vi "Load by Identifier.vi"(8 "error in (no error)":errorcluster, 10 "Identifier":string, 11 "InMemoryUserProvider in":refnum<class "InMemoryUserProvider.lvclass">) -> (0 "error out":errorcluster, 2 "User":refnum<class "User.lvclass">, 3 "InMemoryUserProvider out":refnum<class "InMemoryUserProvider.lvclass">)   [LabVIEW 2020, in "HTTP Server.lvlib" / "InMemoryUserProvider.lvclass"]
uses:
  InMemoryUserProvider.lvclass
  InMemoryUserProvider.lvclass/InMemoryUserProvider.ctl
  User/User.lvclass
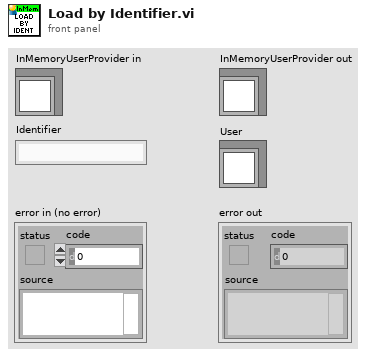
[diagram p1: front panel]
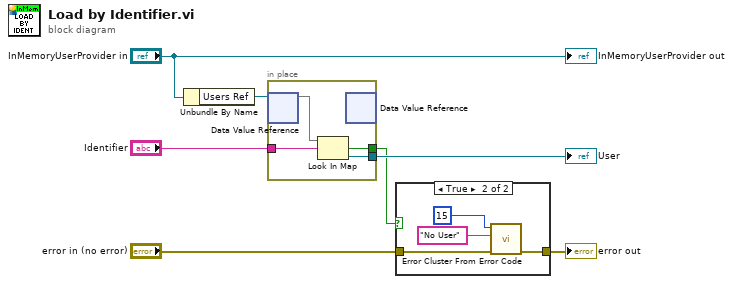
[diagram p0: block diagram]
diagram:
  n1 = Unbundle By Name("InMemoryUserProvider in") -> ("Users Ref"=w7:refnum<data-value>)
  n2 = in-place {
    in-place-border: "Identifier" -> [w10]
    in-place-border: [w9] -> w4
    in-place-border: [w8] -> w2
    n3 = in-place-dvr #1(w7) -> (w11:map{string, refnum<class "User.lvclass">})  [unwired: 1 out]
    n4 = Look In Map(map=w11, key=w10) -> (key not found?=w8:bool, value=w9:refnum<class "User.lvclass">)  [unwired: 1 in]
    n5 = in-place-dvr #1() -> ()  [unwired: 1 in, 2 out]
  }
  "User" <- w4
  n6 = case shown="True" w2 {
    tunnel: "error in (no error)" -> [w12 w14]
    tunnel: [w12 w13] -> w1
    frame False {
    }
    frame True {
      n7 = call <vilib>:"Error Cluster From Error Code.vi"("error in (no error)"=w14, "error message (\"\")"="No User" ("error message (\"\")"), "error code (0)"=15) -> ("error out"=w13:errorcluster)  [unwired: 6 in]
    }
  }
  "error out" <- w1
  "InMemoryUserProvider out" <- "InMemoryUserProvider in"
